vi "HOST_0505.vi"() -> ()   [LabVIEW 2018]
uses:
  <vilib>/rvi/interface/nirviMethod/nirviMethod.xnode
  <vilib>/FPGAPlugInAG/Dynamic/niLvFpga_Reset_Dynamic.vi
  <vilib>/FPGAPlugInAG/Dynamic/niLvFpga_Run_Dynamic.vi
  <vilib>/rvi/interface/nirviOpenFPGA/nirviOpenFPGA.xnode
  <vilib>/rvi/interface/nirviReadWriteControl/nirviReadWriteControl.xnode
  NiFpgaLv.dll
  <vilib>/Utility/error.llb/Error Cluster From Error Code.vi
  <vilib>/rvi/interface/Simulation/niFpgaSimulationCallBeginRW.vi
  <vilib>/rvi/errors/niLvFpgaAdjustHostInterfaceError.vi
  <vilib>/rvi/interface/nirviCloseFPGA/nirviCloseFPGA.xnode
  <instrlib>/niDCPower/nidcpower.llb/niDCPower Measurement Type.ctl
  <vilib>/FPGAPlugInAG/Dynamic/niLvFpga_ReadFifo_Dynamic.vi
  <vilib>/rvi/errors/niLvFpgaMergeErrorWithErrorCode.vi
  <vilib>/FPGAPlugInAG/Dynamic/niLvFpga_Close_Dynamic.vi
  FPGA Bitfiles/GMAX0505_FPGATarget_Target0505_42rFBjRCR8s.lvbitx
  <vilib>/FPGAPlugInAG/PXI-7953R/niLvFpga_Open_PXI-7953R.vi
  <vilib>/rvi/interface/common/dynamic/niFpgaDynamicAddResources.vi
  <vilib>/userdefined/High Color/nirio_resource_hc.ctl
panel:
  out "Прочитали":u8[](array[numeric])
  out "Регистры":bool[](array[boolean])
  in  "Регистры":u8[](array[numeric])=[35, 5, 0, 244, 1, 0, 1, 0, 0, 0, 0, 0, 34, 20, 1, 0, 0, 7, 0, 4, 0, 0, 20, 0, 0, 0, 0, 0, 0, 0, 0, 0, 0, 0, 0, 0, 0, 0, 0, 0, 0, 0, 0, 0, 0, 0, 0, 0, 0, 0, 0, 0, 0, 0, 0, 0, 0, 0, 0, 0, 0, 0, 0, 0, 0, 0, 0, 0, 0, 0, 0, 0, 0, 0, 0, 0, 0, 0, 0, 0, 0, 0, 0, 50, 20, 0, 0, 6, 2, 2, 4, 4, 0, 32, 35, 1, 196, 53, 203, 59, 53, 252, 255, 255, 255, 255, 255, 255, 255, 255, 52, 216, 16, 79, 61, 0, 8, 144, 192, 29, 9, 196, 50, 75, 91, 5, 208, 160, 195, 68, 2, 16, 112, 67, 14, 48, 208, 240, 208, 68, 7, 208, 192, 195, 68, 52, 240, 128, 195, 255, 75, 164, 161, 64, 14, 65, 252, 31, 129, 12, 124, 0, 24, 27, 1, 0, 2, 0, 5, 0, 0, 0, 7, 208, 192, 195, 68, 0, 1, 3, 0, 0, 0, 0, 0, 0, 0, 0, 0, 0, 0, 0, 0, 0, 0, 0, 0, 0, 0, 0, 0, 0, 176, 0, 27, 33, 128, 247, 131, 128, 165, 204, 119, 243, 221, 13, 211, 0, 0, 28, 176, 13, 254, 98, 193, 31, 138, 202, 231, 168, 60, 138, 254, 130, 52, 127, 193, 32, 2, 0, 0, 0, 0, 0, 0, 0, 0, 0, 0, 0, 0, 0, 0, 0, 0, 0]
  out "Записали адресов":u32
  out "世男":bool
  out "Data":u64[][](array[numeric])
  out "Image":T1(plugin-control)
  in  "Период опроса, мс":u32=1
  in  "3,3V_LVDS, V":dbl=3.3 caption="voltage level" format="%_6p"
  in  "3,3V_LVDS_curlim":dbl=0.2 caption="current limit" format="%_6p"
  out "3,3V_LVDS_char":dbl(graph)=1.5967060684808935e-06
  in  "VDDPIX, V":dbl=3.6 caption="voltage level" format="%_6p"
  in  "VDDPIX_curlim":dbl=0.3 caption="current limit" format="%_6p"
  out "VDDPIX_char":dbl(graph)=1.5967060684808935e-06
  in  "VG_RSTH, V":dbl=4.1 caption="voltage level" format="%_6p"
  in  "VG_RSTH_curlim":dbl=0.1 caption="current limit" format="%_6p"
  out "VG_RSTH_char":dbl(graph)=1.5967060684808935e-06
  in  "LED, V":dbl=-3.0 caption="voltage level" format="%_6p"
  in  "LED_curlim":dbl=0.05 caption="current limit" format="%_6p"
  out "LED_char":dbl(graph)=1.5967060684808935e-06
  in  "VDD33A, V":dbl=3.3 caption="voltage level" format="%_6p"
  in  "VDD33A_curlim":dbl=0.3 caption="current limit" format="%_6p"
  out "VDD33A_char":dbl(graph)=1.5967060684808935e-06
  in  "W(T)/R(F)":bool
  in  "Автомат":bool
  in  "VTXH, V":dbl=3.6 caption="voltage level" format="%_6p"
  in  "VDDIO, V":dbl=3.3 caption="voltage level" format="%_6p"
  in  "VDDCL, V":dbl=0.7 caption="voltage level" format="%_6p"
  in  "VDD13, V":dbl=1.3 caption="voltage level" format="%_6p"
  in  "VTXH_curlim":dbl=0.2 caption="current limit" format="%_6p"
  in  "VGRSTL_curlim":dbl=0.1 caption="current limit" format="%_6p"
  in  "VDDIO_curlim":dbl=0.1 caption="current limit" format="%_6p"
  in  "VDDCL_curlim":dbl=0.1 caption="current limit" format="%_6p"
  in  "VTXL_curlim":dbl=0.1 caption="current limit" format="%_6p"
  in  "VDD13_curlim":dbl=1.0 caption="current limit" format="%_6p"
  in  "VGRSTL, V":dbl=-1.3 caption="voltage level" format="%_6p"
  in  "VTXL, V":dbl=-1.3 caption="voltage level" format="%_6p"
  out "VTXH_char":dbl(graph)=-0.007753012065680951
  out "VGRSTL_char":dbl(graph)=6.909391540672134e-05
  out "VDDIO_char":dbl(graph)=9.424895165128459e-05
  out "VDDCL_char":dbl(graph)=-9.950040532110056e-06
  out "VTXL_char":dbl(graph)=9.067752968783287e-05
  out "VDD13_char":dbl(graph)=1.5967060684808935e-06
  in  "VDDPIX_selcur":dbl=0.2 caption="current limit" format="%_6p"
  in  "VDD33A_selcur":dbl=0.2 caption="current limit" format="%_6p"
  in  "VDD13_selcur":dbl=0.75 caption="current limit" format="%_6p"
  in  "VTXL_selcur":dbl=0.09 caption="current limit" format="%_6p"
  out "VDDCL_cur":dbl caption="measurement" format="%_6g"
  out "VTXL_cur":dbl caption="measurement" format="%_6g"
  out "VDD13_cur":dbl caption="measurement" format="%_6g"
  out "VDD33A_cur":dbl caption="measurement" format="%_6g"
  in  "SEL_Time, ms":u32=100
  in  "VG_RSTH_selcur":dbl=0.05 caption="current limit" format="%_6p"
  in  "VTXH_selcur":dbl=0.1 caption="current limit" format="%_6p"
  in  "VGRSTL_selcur":dbl=0.03 caption="current limit" format="%_6p"
  in  "VDDIO_selcur":dbl=0.03 caption="current limit" format="%_6p"
  in  "VDDCL_selcur":dbl=0.02 caption="current limit" format="%_6p"
  out "VDDPIX_cur":dbl caption="measurement" format="%_6g"
  out "VDDIO_cur":dbl caption="measurement" format="%_6g"
  out "VGRSTL_cur":dbl caption="measurement" format="%_6g"
  out "VTXH_cur":dbl caption="measurement" format="%_6g"
  out "VG_RSTH_cur":dbl caption="measurement" format="%_6g"
  out "VDDPIX":u16
  out "VDDPIX":bool
  out "VDD33A":u16
  out "VDD33A":bool
  out "VDD13":u16
  out "VDD13":bool
  out "VTXL":u16
  out "VTXL":bool
  in  "3":refnum<k15>="0" caption="1"
  in  "Проверка сбоев":bool
  out "SEU":bool
  out "SEU":u16
  in  "SPI":bool
  out "REG":bool
  in  "MOVIE":bool
  in  "FRAME!":bool
  in  "SYS_RESET_N":bool
  out "SEL":bool
  in  "SIM_SEL":bool
  out "VG_RSTH":u16
  out "VDDCL":u16
  out "VTXH":u16
  out "VDDIO":u16
  out "VGRSTL":u16
  out "VG_RSTH":bool
  out "VDDCL":bool
  out "VTXH":bool
  out "VDDIO":bool
  out "VGRSTL":bool
  in  "Стоп":bool
  in  "Питание":bool
  in  "LED":bool caption="output enabled"
  in  "0":refnum<k15>="0" caption="1"
  in  "1":refnum<k15>="0"
  in  "2":refnum<k15>="0" caption="1"
  in  "resource name 2":T2="PXI1Slot9"
  in  "SEU":path=path "C:/VPL/LabView/GSENSE2020BSI/SEU"
  in  "SEL":path=path "C:/VPL/LabView/GSENSE2020BSI/SEL"
  out "Номер образца":string="1"
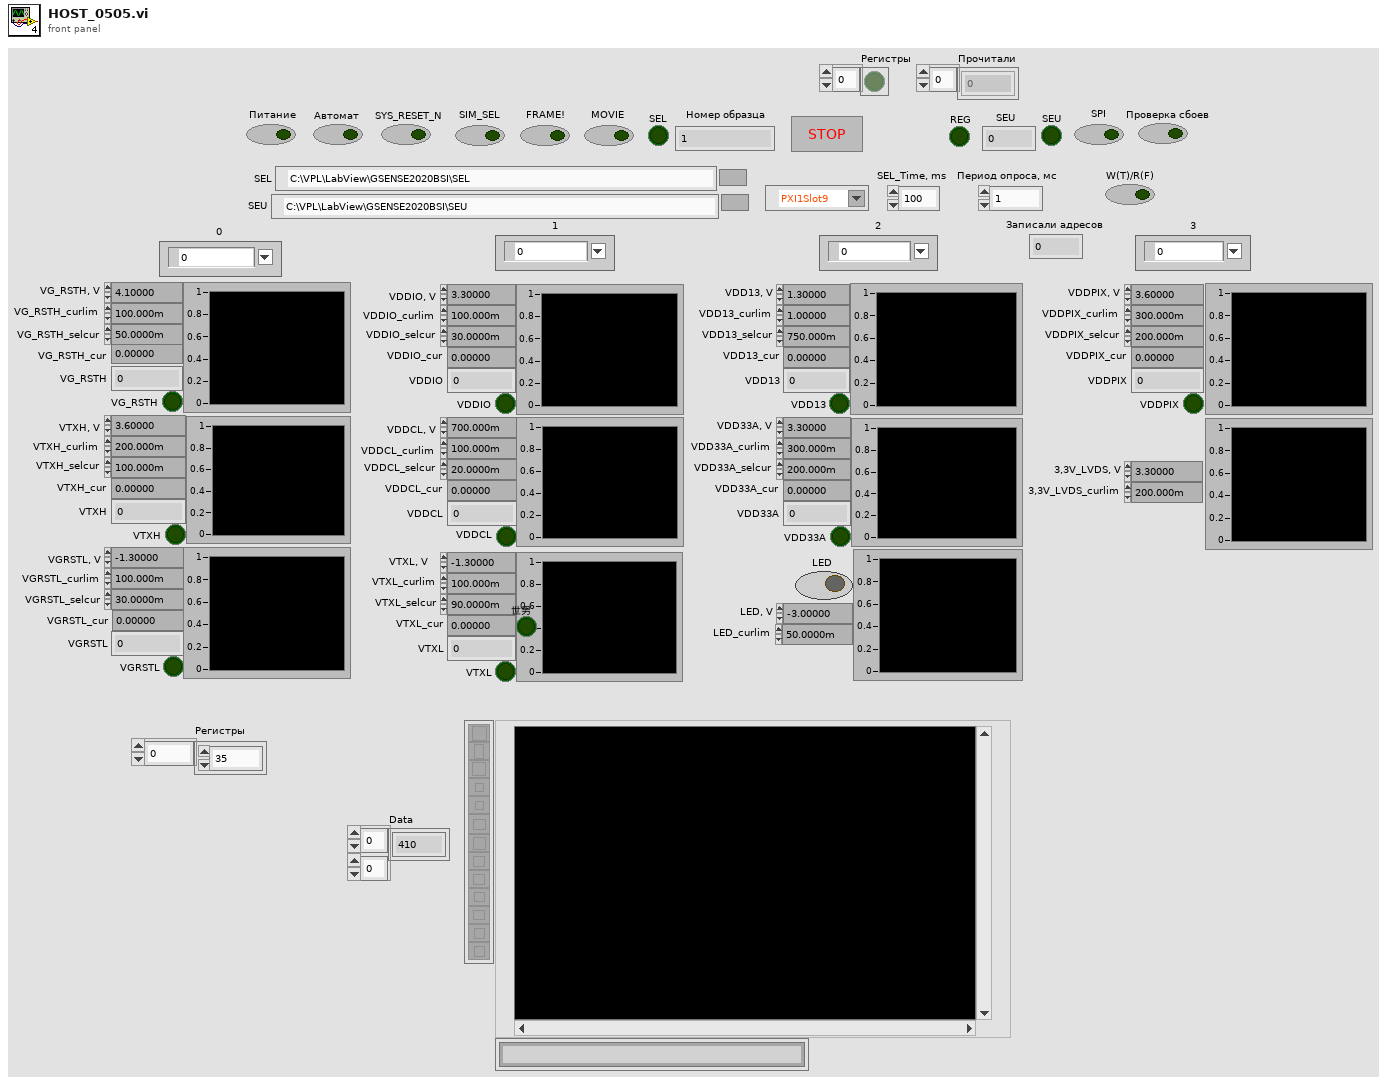
[diagram p1: front panel]
types:
  T1 = typedef "IMAQ Image.ctl" = refnum<image>
  T2 = typedef "nirio_resource_hc.ctl" = tag
  T3 = typedef "Image Type" = u32
  T4 = enum16{"open", "replace", "create", "open or create", "replace or create", "replace or create with confirmation"}
  T5 = typedef "niDCPower Measurement Type.ctl" = i32
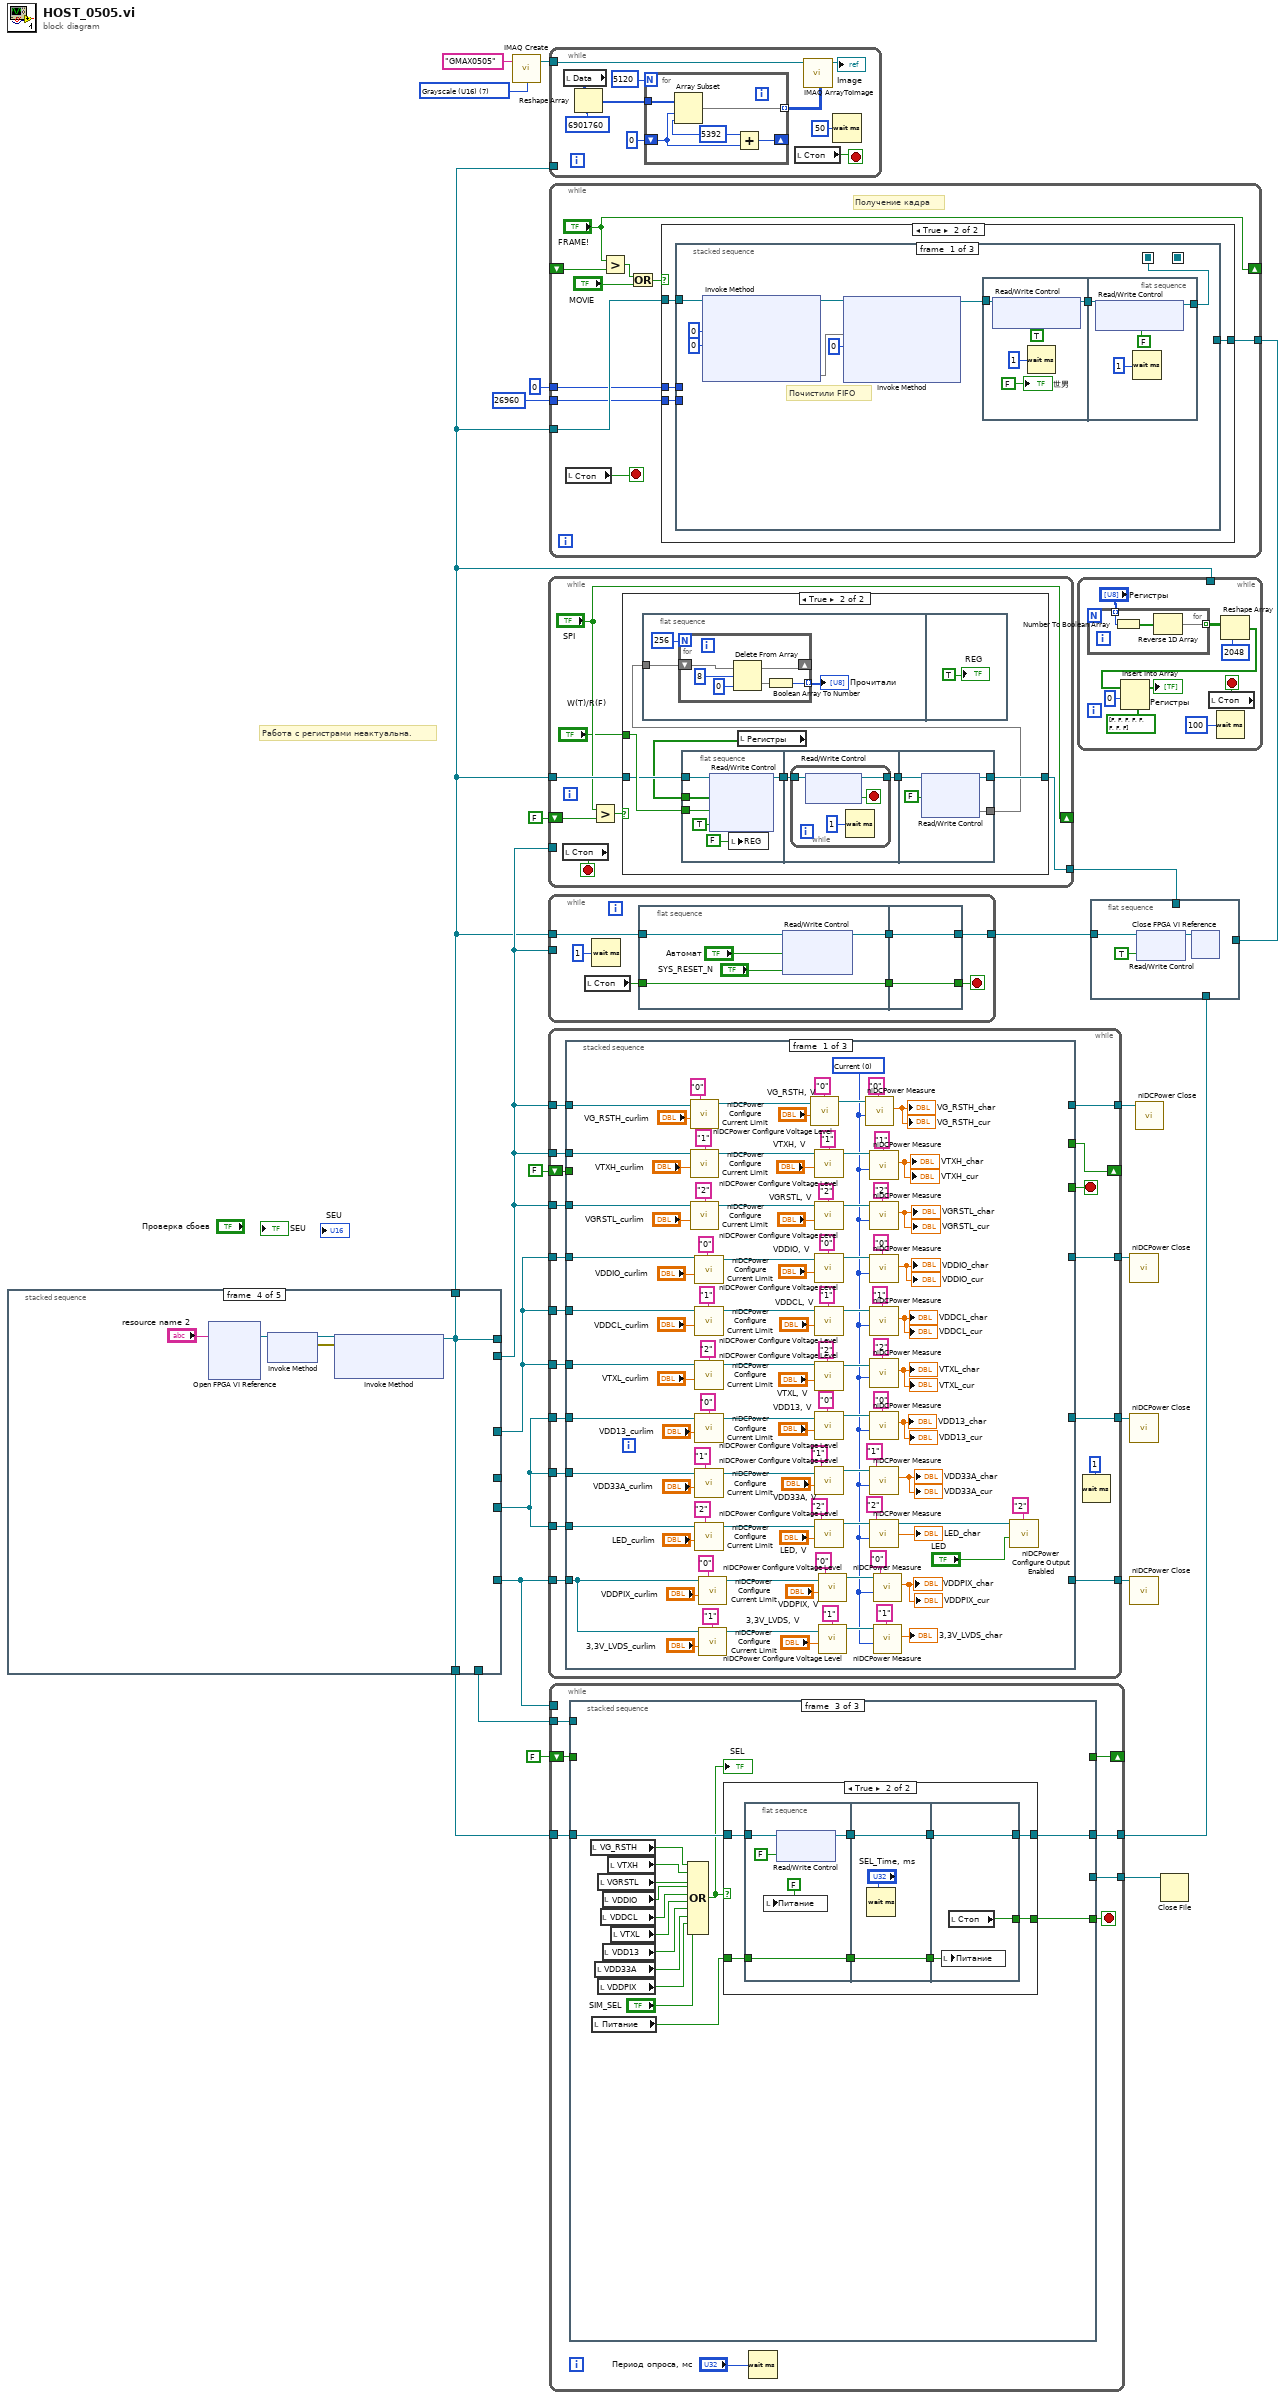
[diagram p0: block diagram]
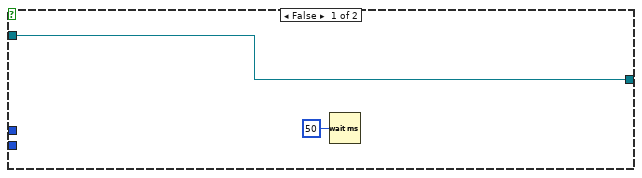
[diagram p2: hidden frame]
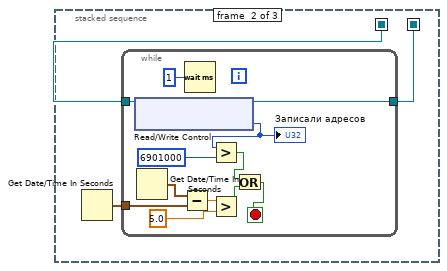
[diagram p3: hidden frame]
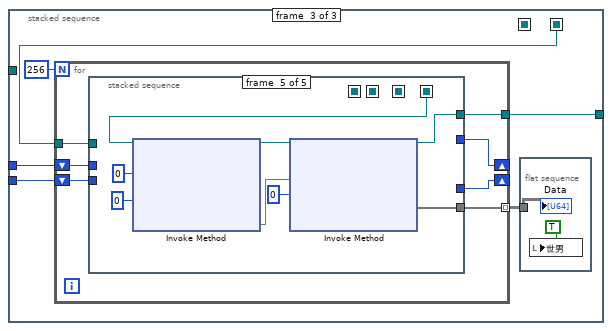
[diagram p4: hidden frame]
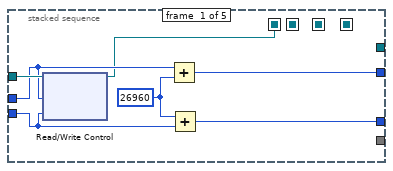
[diagram p5: hidden frame]
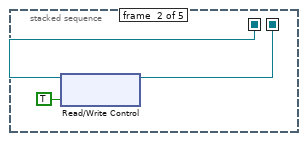
[diagram p6: hidden frame]
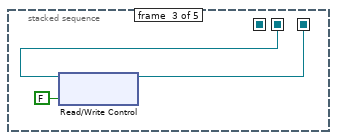
[diagram p7: hidden frame]
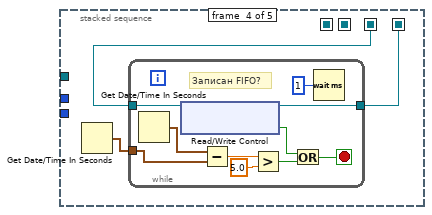
[diagram p8: hidden frame]
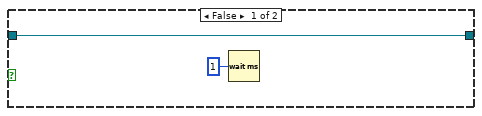
[diagram p9: hidden frame]
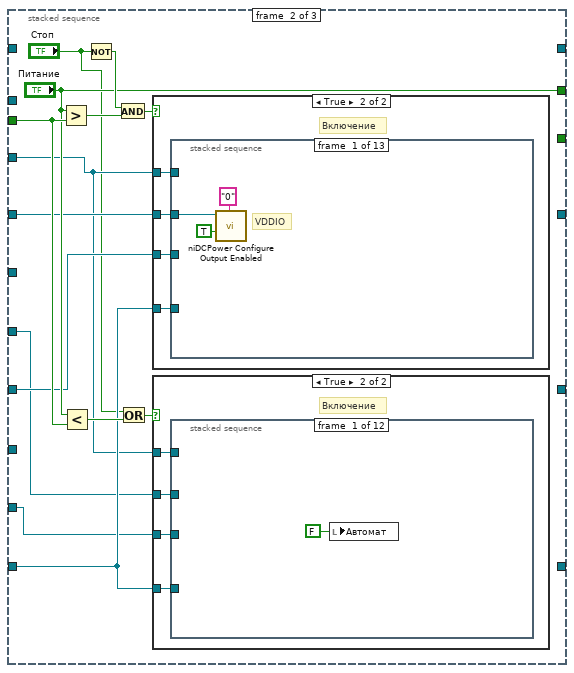
[diagram p10: hidden frame]
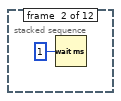
[diagram p12: hidden frame]
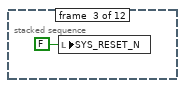
[diagram p13: hidden frame]
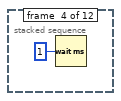
[diagram p14: hidden frame]
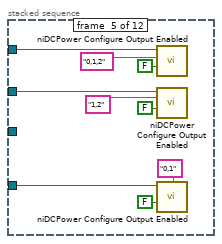
[diagram p15: hidden frame]
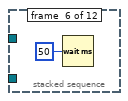
[diagram p16: hidden frame]
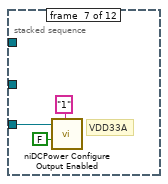
[diagram p17: hidden frame]
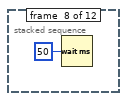
[diagram p18: hidden frame]
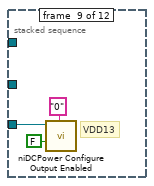
[diagram p19: hidden frame]
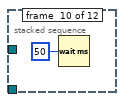
[diagram p20: hidden frame]
diagram:
  w9 = T3 7 items=["Grayscale (U8)", "Grayscale (I16)", "Grayscale (SGL)", "Complex (CSG)", "RGB (U32)", "HSL (U32)", "RGB (U64)", "Grayscale (U16)"] ("Image Type")
  # "Работа с регистрами неактуальна."
  n1 = stacked-sequence {
    tunnel: [_ _ _ _ w109] -> w17
    tunnel: [_ _ _ _ w102] -> w11
    tunnel: [_ _ _ _ w113] -> w18
    tunnel: [_ _ _ w99 _] -> w1
    tunnel: [_ _ _ w99 _] -> w21
    tunnel: [_ w36 _ _ _] -> w22
    tunnel: [_ _ w66 _ _] -> _
    tunnel: [_ _ _ w99 _] -> _
    tunnel: [_ _ _ _ w103] -> w19
    frame #0 {
      w25 = FALSE ("Стоп")
      w27 = FALSE ("Стоп")
      w28 = u16 0 ("ADC")
      # "Обнуление"
      n2 = call "Begin.vi"() -> ("Номер образца 2"=→"Номер образца":string)  [unwired: 11 in]
      n3 = local write "VTXH"(w25) -> ()
      n4 = local write "SIM_SEL"(w25) -> ()
      n5 = local write "SPI"(w25) -> ()
      n6 = local write "Проверка сбоев"(w25) -> ()
      n7 = local write "SEL"(w25) -> ()
      n8 = local write "REG"(w25) -> ()
      n9 = local write "SEU"(w28) -> ()
      n10 = local write "VTXH"(w28) -> ()
      n11 = local write "VDDCL"(w28) -> ()
      n12 = local write "VG_RSTH"(w28) -> ()
      n13 = local write "VDDIO"(w28) -> ()
      n14 = local write "VGRSTL"(w28) -> ()
      n15 = local write "SEU"(w27) -> ()
      n16 = local write "SYS_RESET_N"(w27) -> ()
      n17 = local write "Стоп"(w27) -> ()
      n18 = local write "Питание"(w27) -> ()
      n19 = local write "FRAME!"(w27) -> ()
      n20 = local write "MOVIE"(w27) -> ()
      n21 = local write "LED"(w27) -> ()
      n22 = local write "VG_RSTH"(w27) -> ()
      n23 = local write "VDDCL"(w27) -> ()
      n24 = local write "VGRSTL"(w27) -> ()
      n25 = local write "VDDIO"(w27) -> ()
    }
    frame #1 {
      w31 = "\t"
      # "Лог по токам"
      n26 = local read "Номер образца"() -> (w58:string)
      n27 = Build Path(base path="SEL", name or relative path=w58) -> (appended path=w55:path)
      n28 = Get Date/Time In Seconds() -> (seconds since 1Jan1904=w52:timestamp)
      n29 = call <vilib>:"Check if File or Folder Exists.vi"("path"=w55) -> ("file or folder exists?"=w56:bool, "dup path"=w57:path)  [unwired: 8 in, 1 out]
      n30 = Format Date/Time String(time format string (%c)="%d %H.%M.%S", seconds (now)=w52) -> (date/time string=w50:string)  [unwired: 1 in]
      n31 = case shown="False" w56 {
        tunnel: w57 -> [w64 w65]
        tunnel: [w63 w65] -> w30
        frame False {
          n32 = Create Folder(path (use dialog)=w64) -> (created path=w63:path)  [unwired: 2 in, 2 out]
        }
        frame True {
        }
      }
      n33 = Concatenate Strings(w50, ".xls" ("string")) -> (w49:string)
      n34 = Build Path(base path=w30, name or relative path=w49) -> (appended path=w51:path)
      n35 = Open/Create/Replace File(file path (use dialog)=w51, operation (0:open)=T4."open or create", access (0:read/write)=enum16{"read/write", "read-only", "write-only"}."read/write") -> (refnum out=w53:refnum<file>)  [unwired: 3 in, 2 out]
      n36 = case shown="True" TRUE {
        tunnel: w53 -> [w59 w62]
        tunnel: [w59 w60] -> w48
        frame False {
        }
        frame True {
          n37 = Set File Position(refnum=w62, from (0:start)=enum16{"start", "end", "current"}."end") -> (refnum out=w60:refnum<file>)  [unwired: 2 in, 1 out]
        }
      }
      n38 = Format Into String(initial string=w48, "Time" ("input 1"), w31, "VG_RSTH_cur", w31, "VTXH_cur", w31, "VGRSTL_cur", w31, "VDDIO_cur", w31, "VDDCL_cur", w31, "VTXL_cur", w31, "VDD13_cur", w31, "VDD33A_cur", w31, "VDDPIX_cur", w31, "\r\n") -> (resulting string=w36:refnum<file>)  [unwired: 2 in, 1 out]
    }
    frame #2 {
      w69 = "\t"
      # "Лог по сбоям"
      n39 = local read "Номер образца"() -> (w73:string)
      n40 = Build Path(base path="SEU", name or relative path=w73) -> (appended path=w87:path)
      n41 = Get Date/Time In Seconds() -> (seconds since 1Jan1904=w85:timestamp)
      n42 = call <vilib>:"Check if File or Folder Exists.vi"("path"=w87) -> ("file or folder exists?"=w88:bool, "dup path"=w89:path)  [unwired: 8 in, 1 out]
      n43 = Format Date/Time String(time format string (%c)="%d %H.%M.%S", seconds (now)=w85) -> (date/time string=w83:string)  [unwired: 1 in]
      n44 = case shown="False" w88 {
        tunnel: w89 -> [w95 w96]
        tunnel: [w94 w96] -> w74
        frame False {
          n45 = Create Folder(path (use dialog)=w95) -> (created path=w94:path)  [unwired: 2 in, 2 out]
        }
        frame True {
        }
      }
      n46 = Concatenate Strings(w83, ".xls" ("string")) -> (w82:string)
      n47 = Build Path(base path=w74, name or relative path=w82) -> (appended path=w84:path)
      n48 = Open/Create/Replace File(file path (use dialog)=w84, operation (0:open)=T4."open or create", access (0:read/write)=enum16{"read/write", "read-only", "write-only"}."read/write") -> (refnum out=w86:refnum<file>)  [unwired: 3 in, 2 out]
      n49 = case shown="True" TRUE {
        tunnel: w86 -> [w90 w93]
        tunnel: [w90 w91] -> w81
        frame False {
        }
        frame True {
          n50 = Set File Position(refnum=w93, from (0:start)=enum16{"start", "end", "current"}."end") -> (refnum out=w91:refnum<file>)  [unwired: 2 in, 1 out]
        }
      }
      n51 = Format Into String(initial string=w81, "Time" ("input 1"), w69, "Регистр №" ("input 3"), w69, "Содержание" ("input 4"), w69, "Кол-во сбоев" ("input 7"), "\r\n") -> (resulting string=w66:refnum<file>)  [unwired: 2 in, 1 out]
    }
    frame #3 {
      n52 = xnode "Open FPGA VI Reference"("resource name"="resource name 2") -> ("FPGA VI Reference Out"=w97:refnum<k20>)  [unwired: 1 in, 1 out]
      n53 = xnode "Invoke Method"("FPGA VI Reference In"=w97) -> ("FPGA VI Reference Out"=w101:refnum<k20>, "error out"=w100:errorcluster)  [unwired: 1 in]
      n54 = xnode "Invoke Method"("FPGA VI Reference In"=w101, "error in"=w100) -> ("FPGA VI Reference Out"=w99:refnum<k20>)  [unwired: 1 in, 1 out]
    }
    frame #4 {
      n55 = call <instrlib>:"niDCPower Initialize.vi"("resource name"="2") -> ("error out"=w119:errorcluster, "instrument handle out"=w116:refnum<k15>)  [unwired: 3 in, 6 out]
      n56 = call <instrlib>:"niDCPower Initialize.vi"("resource name"="1") -> ("error out"=w117:errorcluster, "instrument handle out"=w114:refnum<k15>)  [unwired: 3 in, 6 out]
      n57 = call <instrlib>:"niDCPower Initialize.vi"("resource name"="3") -> ("error out"=w107:errorcluster, "instrument handle out"=w108:refnum<k15>)  [unwired: 3 in, 6 out]
      n58 = call <instrlib>:"niDCPower Initialize.vi"("resource name"="0") -> ("error out"=w118:errorcluster, "instrument handle out"=w115:refnum<k15>)  [unwired: 3 in, 6 out]
      n59 = call <instrlib>:"niDCPower Configure Voltage Level.vi"("error in (no error)"=w119, "voltage level"=0.0, "channel name"="0,1,2", "instrument handle"=w116) -> ("instrument handle out"=w109:refnum<k15>)  [unwired: 6 in, 1 out]
      n60 = call <instrlib>:"niDCPower Configure Voltage Level.vi"("error in (no error)"=w117, "voltage level"=0.0, "channel name"="0,1,2", "instrument handle"=w114) -> ("instrument handle out"=w113:refnum<k15>)  [unwired: 6 in, 1 out]
      n61 = call <instrlib>:"niDCPower Configure Voltage Level.vi"("error in (no error)"=w107, "voltage level"=0.0, "channel name"="0,1", "instrument handle"=w108) -> ("instrument handle out"=w103:refnum<k15>)  [unwired: 6 in, 1 out]
      n62 = call <instrlib>:"niDCPower Configure Voltage Level.vi"("error in (no error)"=w118, "voltage level"=0.0, "channel name"="0,1,2", "instrument handle"=w115) -> ("instrument handle out"=w102:refnum<k15>)  [unwired: 6 in, 1 out]
    }
  }
  n63 = call "IMAQ Create"("Image Name"="GMAX0505", "Image Type"=w9) -> ("New Image"=w10:T1)  [unwired: 3 in, 1 out]
  n64 = while {
    tunnel: w1 -> [w129]
    shift-right: ["SPI"] -> _
    shift-left: FALSE ("SPI") -> [w131]
    tunnel: w11 -> [_]
    tunnel: [w127] -> w4
    stop <- w132 stop-if-true
    n65 = local read "Стоп"() -> (w132:bool)
    n66 = Greater?(x="SPI", y=w131) -> (0:w130:bool)
    n67 = case shown="True" w130 {
      tunnel: w129 -> [w133 w139]
      tunnel: [w133 w140] -> w127
      tunnel: "W(T)/R(F)" -> [_ w141]
      frame False {
        n68 = Wait (ms)(milliseconds to wait=u32 1) -> ()  [unwired: 1 out]
      }
      frame True {
        n69 = flat-sequence {
          tunnel: w135 -> [w160]
          frame #0 {
            n70 = for {
              N: 256 -> [_]
              shift-right: [w163] -> _
              shift-left: w160 -> [w166]
              tunnel: [w161] -> w158 mode=indexing
              n71 = Delete From Array(array=w166, length=8, index=0) -> (deleted portion=w162, array with subset deleted=w163)
              n72 = Boolean Array To Number(Boolean array=w162) -> (number=w161:u8)
            }
            "Прочитали" <- w158
          }
          frame #1 {
            "REG" <- TRUE ("REG")
          }
        }
        n73 = flat-sequence {
          tunnel: [w146] -> w138
          tunnel: w141 -> [w145]
          tunnel: w139 -> [w144]
          tunnel: w136 -> [w142]
          tunnel: w138 -> [w149]
          tunnel: [w148] -> w137
          tunnel: w137 -> [w157]
          tunnel: [w155] -> w140
          tunnel: [w154] -> w135
          frame #0 {
            n74 = xnode "Read/Write Control"("FPGA VI Reference In"=w144, "SPI_IN"=w142, "W(T)/R(F)"=w145, "SPI"=TRUE) -> ("FPGA VI Reference Out"=w146:refnum<k20>)  [unwired: 1 in, 1 out]
            n75 = local write "REG"(FALSE ("REG")) -> ()
          }
          frame #1 {
            n76 = while {
              tunnel: w149 -> [w153]
              tunnel: [w150] -> w148
              stop <- w152 stop-if-true
              n77 = xnode "Read/Write Control"("FPGA VI Reference In"=w153) -> ("FPGA VI Reference Out"=w150:refnum<k20>, "SPI_OFF"=w152:bool)  [unwired: 1 in, 1 out]
              n78 = Wait (ms)(milliseconds to wait=u32 1) -> ()  [unwired: 1 out]
            }
          }
          frame #2 {
            n79 = xnode "Read/Write Control"("FPGA VI Reference In"=w157, "SPI"=FALSE) -> ("FPGA VI Reference Out"=w155:refnum<k20>, "SPI_OUT"=w154)  [unwired: 1 in, 1 out]
          }
        }
        n80 = local read "Регистры"() -> (w136:bool[])
      }
    }
  }
  n81 = while {
    tunnel: w1 -> [w173]
    tunnel: [w172] -> w2
    tunnel: w11 -> [_]
    stop <- w168 stop-if-true
    n82 = local read "Стоп"() -> (w169:bool)
    n83 = Wait (ms)(milliseconds to wait=u32 1) -> ()  [unwired: 1 out]
    n84 = flat-sequence {
      tunnel: w173 -> [w179]
      tunnel: [w178] -> w171
      tunnel: [w177] -> w170
      tunnel: w169 -> [w177]
      tunnel: [w181] -> w172
      tunnel: w171 -> [w181]
      tunnel: w170 -> [w180]
      tunnel: [w180] -> w168
      frame #0 {
        n85 = xnode "Read/Write Control"("FPGA VI Reference In"=w179, "Автомат"="Автомат", "SYS_RST_N"="SYS_RESET_N") -> ("FPGA VI Reference Out"=w178:refnum<k20>)  [unwired: 1 in, 1 out]
      }
      frame #1 {
      }
    }
  }
  n86 = while {
    shift-right: [w198] -> _
    shift-left: FALSE -> [w199]
    tunnel: w11 -> [w197]
    tunnel: w18 -> [w191]
    tunnel: w17 -> [w188]
    tunnel: w19 -> [w196]
    tunnel: w11 -> [w193]
    tunnel: w11 -> [w192]
    tunnel: w18 -> [w190]
    tunnel: w18 -> [w189]
    tunnel: w17 -> [w187]
    tunnel: w17 -> [w186]
    tunnel: [w185] -> w16
    tunnel: [w184] -> w15
    tunnel: [w183] -> w14
    tunnel: [w182] -> w13
    stop <- w195 stop-if-true
    n87 = stacked-sequence {
      tunnel: w199 -> [_ w315 _]
      tunnel: [_ "Питание" _] -> w198
      tunnel: w197 -> [w211 _ w379]
      tunnel: w196 -> [w200 w306 w376]
      tunnel: [_ _ w380] -> w195
      tunnel: w193 -> [w210 _ _]
      tunnel: w192 -> [w209 w303 _]
      tunnel: w191 -> [w208 w309 w378]
      tunnel: w190 -> [w207 _ _]
      tunnel: w189 -> [w206 w304 _]
      tunnel: w188 -> [w205 w308 w377]
      tunnel: w187 -> [w204 _ _]
      tunnel: w186 -> [w203 w305 _]
      tunnel: [_ _ w379] -> w185
      tunnel: [_ _ w378] -> w184
      tunnel: [_ _ w377] -> w183
      tunnel: [_ _ w376] -> w182
      frame #0 {
        w225 = T5 0 items=["Current", "Voltage"] ("measurement type")
        n88 = call <instrlib>:"niDCPower Configure Current Limit.vi"("current limit"="VG_RSTH_curlim", "channel name"="0", "instrument handle"=w211) -> ("instrument handle out"=w242:refnum<k15>)  [unwired: 7 in, 1 out]
        n89 = call <instrlib>:"niDCPower Configure Current Limit.vi"("current limit"="VTXH_curlim", "channel name"="1", "instrument handle"=w210) -> ("instrument handle out"=w282:refnum<k15>)  [unwired: 7 in, 1 out]
        n90 = call <instrlib>:"niDCPower Configure Current Limit.vi"("current limit"="VGRSTL_curlim", "channel name"="2", "instrument handle"=w209) -> ("instrument handle out"=w283:refnum<k15>)  [unwired: 7 in, 1 out]
        n91 = call <instrlib>:"niDCPower Configure Current Limit.vi"("current limit"="VDDIO_curlim", "channel name"="0", "instrument handle"=w208) -> ("instrument handle out"=w284:refnum<k15>)  [unwired: 7 in, 1 out]
        n92 = call <instrlib>:"niDCPower Configure Current Limit.vi"("current limit"="VDDCL_curlim", "channel name"="1", "instrument handle"=w207) -> ("instrument handle out"=w285:refnum<k15>)  [unwired: 7 in, 1 out]
        n93 = call <instrlib>:"niDCPower Configure Current Limit.vi"("current limit"="VTXL_curlim", "channel name"="2", "instrument handle"=w206) -> ("instrument handle out"=w286:refnum<k15>)  [unwired: 7 in, 1 out]
        n94 = call <instrlib>:"niDCPower Configure Current Limit.vi"("current limit"="VDD13_curlim", "channel name"="0", "instrument handle"=w205) -> ("instrument handle out"=w287:refnum<k15>)  [unwired: 7 in, 1 out]
        n95 = call <instrlib>:"niDCPower Configure Current Limit.vi"("current limit"="VDD33A_curlim", "channel name"="1", "instrument handle"=w204) -> ("instrument handle out"=w255:refnum<k15>)  [unwired: 7 in, 1 out]
        n96 = call <instrlib>:"niDCPower Configure Current Limit.vi"("current limit"="LED_curlim", "channel name"="2", "instrument handle"=w203) -> ("instrument handle out"=w250:refnum<k15>)  [unwired: 7 in, 1 out]
        n97 = call <instrlib>:"niDCPower Configure Current Limit.vi"("current limit"="VDDPIX_curlim", "channel name"="0", "instrument handle"=w200) -> ("instrument handle out"=w235:refnum<k15>)  [unwired: 7 in, 1 out]
        n98 = call <instrlib>:"niDCPower Configure Current Limit.vi"("current limit"="3,3V_LVDS_curlim", "channel name"="1", "instrument handle"=w200) -> ("instrument handle out"=w230:refnum<k15>)  [unwired: 7 in, 1 out]
        n99 = call <instrlib>:"niDCPower Configure Voltage Level.vi"("voltage level"="VG_RSTH, V", "channel name"="0", "instrument handle"=w242) -> ("instrument handle out"=w245:refnum<k15>)  [unwired: 7 in, 1 out]
        n100 = call <instrlib>:"niDCPower Configure Voltage Level.vi"("voltage level"="VTXH, V", "channel name"="1", "instrument handle"=w282) -> ("instrument handle out"=w265:refnum<k15>)  [unwired: 7 in, 1 out]
        n101 = call <instrlib>:"niDCPower Configure Voltage Level.vi"("voltage level"="VGRSTL, V", "channel name"="2", "instrument handle"=w283) -> ("instrument handle out"=w264:refnum<k15>)  [unwired: 7 in, 1 out]
        n102 = call <instrlib>:"niDCPower Configure Voltage Level.vi"("voltage level"="VDDIO, V", "channel name"="0", "instrument handle"=w284) -> ("instrument handle out"=w263:refnum<k15>)  [unwired: 7 in, 1 out]
        n103 = call <instrlib>:"niDCPower Configure Voltage Level.vi"("voltage level"="VDDCL, V", "channel name"="1", "instrument handle"=w285) -> ("instrument handle out"=w262:refnum<k15>)  [unwired: 7 in, 1 out]
        n104 = call <instrlib>:"niDCPower Configure Voltage Level.vi"("voltage level"="VTXL, V", "channel name"="2", "instrument handle"=w286) -> ("instrument handle out"=w261:refnum<k15>)  [unwired: 7 in, 1 out]
        n105 = call <instrlib>:"niDCPower Configure Voltage Level.vi"("voltage level"="VDD13, V", "channel name"="0", "instrument handle"=w287) -> ("instrument handle out"=w260:refnum<k15>)  [unwired: 7 in, 1 out]
        n106 = call <instrlib>:"niDCPower Configure Voltage Level.vi"("voltage level"="VDD33A, V", "channel name"="1", "instrument handle"=w255) -> ("instrument handle out"=w258:refnum<k15>)  [unwired: 7 in, 1 out]
        n107 = call <instrlib>:"niDCPower Configure Voltage Level.vi"("voltage level"="LED, V", "channel name"="2", "instrument handle"=w250) -> ("instrument handle out"=w247:refnum<k15>)  [unwired: 7 in, 1 out]
        n108 = call <instrlib>:"niDCPower Configure Voltage Level.vi"("voltage level"="VDDPIX, V", "channel name"="0", "instrument handle"=w235) -> ("instrument handle out"=w238:refnum<k15>)  [unwired: 7 in, 1 out]
        n109 = call <instrlib>:"niDCPower Configure Voltage Level.vi"("voltage level"="3,3V_LVDS, V", "channel name"="1", "instrument handle"=w230) -> ("instrument handle out"=w227:refnum<k15>)  [unwired: 7 in, 1 out]
        n110 = call <instrlib>:"niDCPower Measure.vi"("measurement type"=w225, "channel name"="0", "instrument handle"=w245) -> ("measurement"=→"VG_RSTH_char" →"VG_RSTH_cur":dbl)  [unwired: 6 in, 2 out]
        n111 = call <instrlib>:"niDCPower Measure.vi"("measurement type"=w225, "channel name"="1", "instrument handle"=w265) -> ("measurement"=→"VTXH_char" →"VTXH_cur":dbl)  [unwired: 6 in, 2 out]
        n112 = call <instrlib>:"niDCPower Measure.vi"("measurement type"=w225, "channel name"="2", "instrument handle"=w264) -> ("measurement"=→"VGRSTL_char" →"VGRSTL_cur":dbl)  [unwired: 6 in, 2 out]
        n113 = call <instrlib>:"niDCPower Measure.vi"("measurement type"=w225, "channel name"="0", "instrument handle"=w263) -> ("measurement"=→"VDDIO_char" →"VDDIO_cur":dbl)  [unwired: 6 in, 2 out]
        n114 = call <instrlib>:"niDCPower Measure.vi"("measurement type"=w225, "channel name"="1", "instrument handle"=w262) -> ("measurement"=→"VDDCL_char" →"VDDCL_cur":dbl)  [unwired: 6 in, 2 out]
        n115 = call <instrlib>:"niDCPower Measure.vi"("measurement type"=w225, "channel name"="2", "instrument handle"=w261) -> ("measurement"=→"VTXL_char" →"VTXL_cur":dbl)  [unwired: 6 in, 2 out]
        n116 = call <instrlib>:"niDCPower Measure.vi"("measurement type"=w225, "channel name"="0", "instrument handle"=w260) -> ("measurement"=→"VDD13_char" →"VDD13_cur":dbl)  [unwired: 6 in, 2 out]
        n117 = call <instrlib>:"niDCPower Measure.vi"("measurement type"=w225, "channel name"="1", "instrument handle"=w258) -> ("measurement"=→"VDD33A_char" →"VDD33A_cur":dbl)  [unwired: 6 in, 2 out]
        n118 = call <instrlib>:"niDCPower Measure.vi"("measurement type"=w225, "channel name"="2", "instrument handle"=w247) -> ("measurement"=→"LED_char":dbl, "instrument handle out"=w213:refnum<k15>)  [unwired: 6 in, 1 out]
        n119 = call <instrlib>:"niDCPower Measure.vi"("measurement type"=w225, "channel name"="0", "instrument handle"=w238) -> ("measurement"=→"VDDPIX_char" →"VDDPIX_cur":dbl)  [unwired: 6 in, 2 out]
        n120 = call <instrlib>:"niDCPower Measure.vi"("measurement type"=w225, "channel name"="1", "instrument handle"=w227) -> ("measurement"=→"3,3V_LVDS_char":dbl)  [unwired: 6 in, 2 out]
        n121 = call <instrlib>:"niDCPower Configure Output Enabled.vi"("output enabled"="LED", "channel name"="2", "instrument handle"=w213) -> ()  [unwired: 7 in, 2 out]
      }
      frame #1 {
        n122 = Greater?(x="Питание", y=w315) -> (0:w313:bool)
        n123 = Less?(x="Питание", y=w315) -> (x < y?=w311:bool)
        n124 = Not(x="Стоп") -> (.not. x?=w312:bool)
        n125 = And(x=w312, y=w313) -> (x .and. y?=w314:bool)
        n126 = Or(x="Стоп", y=w311) -> (x .or. y?=w307:bool)
        n127 = case shown="True" w314 {
          tunnel: w309 -> [_ w349]
          tunnel: w308 -> [_ w348]
          tunnel: w303 -> [_ w347]
          tunnel: w306 -> [_ w346]
          frame False {
          }
          frame True {
            # "Включение"
            n128 = stacked-sequence {
              tunnel: w349 -> [w350 _ _ _ _ _ w366 _ _ _ _ _ _]
              tunnel: w348 -> [_ _ w354 _ w358 _ _ _ _ _ _ _ _]
              tunnel: w347 -> [_ _ _ _ _ _ w369 _ _ _ _ _ _]
              tunnel: w346 -> [_ _ _ _ _ _ w365 _ _ _ _ _ _]
              frame #0 {
                # "VDDIO"
                n129 = call <instrlib>:"niDCPower Configure Output Enabled.vi"("output enabled"=TRUE, "channel name"="0", "instrument handle"=w350) -> ()  [unwired: 7 in, 2 out]
              }
              frame #1 {
                n130 = Wait (ms)(milliseconds to wait=u32 50) -> ()  [unwired: 1 out]
              }
              frame #2 {
                # "VDD13"
                n131 = call <instrlib>:"niDCPower Configure Output Enabled.vi"("output enabled"=TRUE, "channel name"="0", "instrument handle"=w354) -> ()  [unwired: 7 in, 2 out]
              }
              frame #3 {
                n132 = Wait (ms)(milliseconds to wait=u32 50) -> ()  [unwired: 1 out]
              }
              frame #4 {
                # "VDD33А"
                n133 = call <instrlib>:"niDCPower Configure Output Enabled.vi"("output enabled"=TRUE, "channel name"="1", "instrument handle"=w358) -> ()  [unwired: 7 in, 2 out]
              }
              frame #5 {
                n134 = Wait (ms)(milliseconds to wait=u32 50) -> ()  [unwired: 1 out]
              }
              frame #6 {
                n135 = call <instrlib>:"niDCPower Configure Output Enabled.vi"("output enabled"=TRUE, "channel name"="0,1,2", "instrument handle"=w369) -> ()  [unwired: 7 in, 2 out]
                n136 = call <instrlib>:"niDCPower Configure Output Enabled.vi"("output enabled"=TRUE, "channel name"="1,2", "instrument handle"=w366) -> ()  [unwired: 7 in, 2 out]
                n137 = call <instrlib>:"niDCPower Configure Output Enabled.vi"("output enabled"=TRUE, "channel name"="0,1", "instrument handle"=w365) -> ()  [unwired: 7 in, 2 out]
              }
              frame #7 {
                n138 = Wait (ms)(milliseconds to wait=u32 50) -> ()  [unwired: 1 out]
              }
              frame #8 {
                n139 = local write "SYS_RESET_N"(TRUE ("SYS_RESET_N")) -> ()
              }
              frame #9 {
                n140 = Wait (ms)(milliseconds to wait=u32 1) -> ()  [unwired: 1 out]
              }
              frame #10 {
                n141 = local write "Автомат"(TRUE ("Автомат")) -> ()
              }
              frame #11 {
                n142 = Wait (ms)(milliseconds to wait=u32 1) -> ()  [unwired: 1 out]
              }
              frame #12 {
                # "Прошиваем регистры"
              }
            }
          }
        }
        n143 = case shown="True" w307 {
          tunnel: w304 -> [_ w319]
          tunnel: w305 -> [_ w318]
          tunnel: w303 -> [_ w317]
          tunnel: w306 -> [_ w316]
          frame False {
          }
          frame True {
            # "Включение"
            n144 = stacked-sequence {
              tunnel: w319 -> [_ _ _ _ w328 _ _ _ _ _ w342 _]
              tunnel: w318 -> [_ _ _ _ _ _ w334 _ w338 _ _ _]
              tunnel: w317 -> [_ _ _ _ w331 _ _ _ _ _ _ _]
              tunnel: w316 -> [_ _ _ _ w327 _ _ _ _ _ _ _]
              frame #0 {
                n145 = local write "Автомат"(FALSE ("Автомат")) -> ()
              }
              frame #1 {
                n146 = Wait (ms)(milliseconds to wait=u32 1) -> ()  [unwired: 1 out]
              }
              frame #2 {
                n147 = local write "SYS_RESET_N"(FALSE ("SYS_RESET_N")) -> ()
              }
              frame #3 {
                n148 = Wait (ms)(milliseconds to wait=u32 1) -> ()  [unwired: 1 out]
              }
              frame #4 {
                n149 = call <instrlib>:"niDCPower Configure Output Enabled.vi"("output enabled"=FALSE, "channel name"="0,1,2", "instrument handle"=w331) -> ()  [unwired: 7 in, 2 out]
                n150 = call <instrlib>:"niDCPower Configure Output Enabled.vi"("output enabled"=FALSE, "channel name"="1,2", "instrument handle"=w328) -> ()  [unwired: 7 in, 2 out]
                n151 = call <instrlib>:"niDCPower Configure Output Enabled.vi"("output enabled"=FALSE, "channel name"="0,1", "instrument handle"=w327) -> ()  [unwired: 7 in, 2 out]
              }
              frame #5 {
                n152 = Wait (ms)(milliseconds to wait=u32 50) -> ()  [unwired: 1 out]
              }
              frame #6 {
                # "VDD33А"
                n153 = call <instrlib>:"niDCPower Configure Output Enabled.vi"("output enabled"=FALSE, "channel name"="1", "instrument handle"=w334) -> ()  [unwired: 7 in, 2 out]
              }
              frame #7 {
                n154 = Wait (ms)(milliseconds to wait=u32 50) -> ()  [unwired: 1 out]
              }
              frame #8 {
                # "VDD13"
                n155 = call <instrlib>:"niDCPower Configure Output Enabled.vi"("output enabled"=FALSE, "channel name"="0", "instrument handle"=w338) -> ()  [unwired: 7 in, 2 out]
              }
              frame #9 {
                n156 = Wait (ms)(milliseconds to wait=u32 50) -> ()  [unwired: 1 out]
              }
              frame #10 {
                # "VDDIO"
                n157 = call <instrlib>:"niDCPower Configure Output Enabled.vi"("output enabled"=FALSE, "channel name"="0", "instrument handle"=w342) -> ()  [unwired: 7 in, 2 out]
              }
              frame #11 {
                n158 = Wait (ms)(milliseconds to wait=u32 50) -> ()  [unwired: 1 out]
              }
            }
          }
        }
      }
      frame #2 {
        n159 = local read "Стоп"() -> (w380:bool)
      }
    }
    n160 = Wait (ms)(milliseconds to wait=u32 1) -> ()  [unwired: 1 out]
  }
  n161 = while {
    tunnel: w10 -> [w387]
    tunnel: w1 -> [_]
    stop <- w390 stop-if-true
    n162 = local read "Data"() -> (w383:u64[][])
    n163 = Reshape Array(w383, 6901760 ("dimension size")) -> (w381:u64[])
    n164 = for {
      N: 5120 ("length 2") -> [_]
      tunnel: w381 -> [w395]
      shift-right: [w394] -> _
      shift-left: 0 ("index") -> [w393]
      tunnel: [w392] -> w385 mode=indexing
      w391 = 5392 ("length")
      n165 = Array Subset(array=w395, index=w393, length=w391) -> (w392:u64[])
      n166 = Add(x=w391, y=w393) -> (x+y=w394:i32)
    }
    n167 = local read "Стоп"() -> (w390:bool)
    n168 = call "IMAQ ArrayToImage"("Image Pixels (U16)"=w385, "Image"=w387) -> ("Image Out"=→"Image":T1)  [unwired: 8 in, 1 out]
    n169 = Wait (ms)(milliseconds to wait=u32 50) -> ()  [unwired: 1 out]
  }
  n170 = while {
    tunnel: w1 -> [w402]
    shift-right: ["FRAME!"] -> _
    shift-left: _ -> [w405]
    tunnel: u32 0 -> [w401]
    tunnel: u32 26960 ("163840") -> [w400]
    tunnel: [w399] -> w3
    stop <- w398 stop-if-true
    # "Получение кадра"
    n171 = local read "Стоп"() -> (w398:bool)
    n172 = Greater?(x="FRAME!", y=w405) -> (0:w404:bool)
    n173 = Or(x=w404, y="MOVIE") -> (x .or. y?=w403:bool)
    n174 = case shown="True" w403 {
      tunnel: w402 -> [w406 w411]
      tunnel: w401 -> [_ w410]
      tunnel: w400 -> [_ w409]
      tunnel: [w406 w408] -> w399
      frame False {
        n175 = Wait (ms)(milliseconds to wait=u32 50) -> ()  [unwired: 1 out]
      }
      frame True {
        n176 = stacked-sequence {
          seq-local: [w413 _ _] -> [_ w431 _]
          seq-local: [_ w430 _] -> [_ _ w446]
          tunnel: w411 -> [w416 _ _]
          tunnel: w410 -> [_ _ w449]
          tunnel: w409 -> [_ _ w448]
          tunnel: [_ _ w445] -> w408
          frame #0 {
            # "Почистили FIFO"
            n177 = xnode "Invoke Method"("FPGA VI Reference In"=w416, "Number of Elements"=u32 0, "Timeout (ms)"=0) -> ("FPGA VI Reference Out"=w415:refnum<k20>, "Elements Remaining"=w417)  [unwired: 1 in, 2 out]
            n178 = xnode "Invoke Method"("FPGA VI Reference In"=w415, "Number of Elements"=w417, "Timeout (ms)"=0) -> ("FPGA VI Reference Out"=w414:refnum<k20>)  [unwired: 1 in, 3 out]
            n179 = flat-sequence {
              tunnel: w414 -> [w425]
              tunnel: [w421] -> w412
              tunnel: [w427] -> w413
              tunnel: w412 -> [w426]
              frame #0 {
                n180 = xnode "Read/Write Control"("FPGA VI Reference In"=w425, "Кадр в память"=TRUE ("EXPOSURE")) -> ("FPGA VI Reference Out"=w421:refnum<k20>)  [unwired: 1 in, 1 out]
                n181 = Wait (ms)(milliseconds to wait=u32 1) -> ()  [unwired: 1 out]
                "世男" <- FALSE
              }
              frame #1 {
                n182 = xnode "Read/Write Control"("FPGA VI Reference In"=w426, "Кадр в память"=FALSE) -> ("FPGA VI Reference Out"=w427:refnum<k20>)  [unwired: 1 in, 1 out]
                n183 = Wait (ms)(milliseconds to wait=u32 1) -> ()  [unwired: 1 out]
              }
            }
          }
          frame #1 {
            n184 = Get Date/Time In Seconds() -> (seconds since 1Jan1904=w432:timestamp)
            n185 = while {
              tunnel: [w443] -> w430
              tunnel: w431 -> [w442]
              tunnel: w432 -> [w439]
              stop <- w434 stop-if-true
              n186 = xnode "Read/Write Control"("FPGA VI Reference In"=w442) -> ("FPGA VI Reference Out"=w443:refnum<k20>, "Записали адресов"=w433:u32)  [unwired: 1 in, 1 out]
              "Записали адресов" <- w433
              n187 = Get Date/Time In Seconds() -> (seconds since 1Jan1904=w440:timestamp)
              n188 = Subtract(x=w440, y=w439) -> (x-y=w438:dbl)
              n189 = Wait (ms)(milliseconds to wait=u32 1) -> ()  [unwired: 1 out]
              n190 = Greater?(x=w433, y=u32 6901000) -> (0:w436:bool)
              n191 = Greater?(x=w438, y=5.0) -> (0:w435:bool)
              n192 = Or(x=w436, y=w435) -> (x .or. y?=w434:bool)
            }
          }
          frame #2 {
            n193 = for {
              N: 256 -> [_]
              tunnel: w446 -> [w459]
              shift-right: [w456] -> _
              shift-left: w449 -> [w458]
              shift-right: [w455] -> _
              shift-left: w448 -> [w457]
              tunnel: [w454] -> w447 mode=indexing
              tunnel: [w453] -> w445
              n194 = stacked-sequence {
                seq-local: [w460 _ _ _ _] -> [_ w468 _ _ _]
                seq-local: [_ w467 _ _ _] -> [_ _ w471 _ _]
                seq-local: [_ _ w470 _ _] -> [_ _ _ w475 _]
                seq-local: [_ _ _ w474 _] -> [_ _ _ _ w486]
                tunnel: w459 -> [w466 _ _ _ _]
                tunnel: w458 -> [w464 _ _ _ _]
                tunnel: w457 -> [w463 _ _ _ _]
                tunnel: [w462 _ _ _ _] -> w456
                tunnel: [w461 _ _ _ _] -> w455
                tunnel: [_ _ _ _ w488] -> w454
                tunnel: [_ _ _ _ w487] -> w453
                frame #0 {
                  w465 = u32 26960 ("163840")
                  n195 = xnode "Read/Write Control"("FPGA VI Reference In"=w466, "Нач_адр"=w464, "Кон_адр"=w463) -> ("FPGA VI Reference Out"=w460:refnum<k20>)  [unwired: 1 in, 1 out]
                  n196 = Add(x=w464, y=w465) -> (x+y=w462:u32)
                  n197 = Add(x=w465, y=w463) -> (x+y=w461:u32)
                }
                frame #1 {
                  n198 = xnode "Read/Write Control"("FPGA VI Reference In"=w468, "Кадр на ПК"=TRUE ("HOST")) -> ("FPGA VI Reference Out"=w467:refnum<k20>)  [unwired: 1 in, 1 out]
                }
                frame #2 {
                  n199 = xnode "Read/Write Control"("FPGA VI Reference In"=w471, "Кадр на ПК"=FALSE ("HOST")) -> ("FPGA VI Reference Out"=w470:refnum<k20>)  [unwired: 1 in, 1 out]
                }
                frame #3 {
                  n200 = Get Date/Time In Seconds() -> (seconds since 1Jan1904=w473:timestamp)
                  n201 = while {
                    tunnel: w475 -> [w484]
                    tunnel: [w483] -> w474
                    tunnel: w473 -> [w481]
                    stop <- w476 stop-if-true
                    # "Записан FIFO?"
                    n202 = Get Date/Time In Seconds() -> (seconds since 1Jan1904=w482:timestamp)
                    n203 = xnode "Read/Write Control"("FPGA VI Reference In"=w484) -> ("FPGA VI Reference Out"=w483:refnum<k20>, "Записали FIFO"=w478:bool)  [unwired: 1 in, 1 out]
                    n204 = Subtract(x=w482, y=w481) -> (x-y=w480:dbl)
                    n205 = Greater?(x=w480, y=5.0) -> (0:w477:bool)
                    n206 = Or(x=w478, y=w477) -> (x .or. y?=w476:bool)
                    n207 = Wait (ms)(milliseconds to wait=u32 1) -> ()  [unwired: 1 out]
                  }
                }
                frame #4 {
                  n208 = xnode "Invoke Method"("FPGA VI Reference In"=w486, "Number of Elements"=u32 0, "Timeout (ms)"=0) -> ("FPGA VI Reference Out"=w492:refnum<k20>, "Elements Remaining"=w493)  [unwired: 1 in, 2 out]
                  n209 = xnode "Invoke Method"("FPGA VI Reference In"=w492, "Number of Elements"=w493, "Timeout (ms)"=0) -> ("FPGA VI Reference Out"=w487:refnum<k20>, "Data"=w488:void[])  [unwired: 1 in, 2 out]
                }
              }
            }
            n210 = flat-sequence {
              tunnel: w447 -> [w451]
              frame #0 {
                n211 = local write "世男"(TRUE) -> ()
                "Data" <- w451
              }
            }
          }
        }
      }
    }
  }
  n212 = while {
    tunnel: w21 -> [w496]
    shift-right: [w500] -> _
    shift-left: FALSE ("Питание") -> [w501]
    tunnel: w22 -> [w498]
    tunnel: [w495] -> w23
    tunnel: [w494] -> w5
    tunnel: w19 -> [_]
    stop <- w497 stop-if-true
    n213 = stacked-sequence {
      tunnel: w501 -> [w504 _ _]
      tunnel: [w503 _ _] -> w500
      tunnel: w498 -> [_ w605 _]
      tunnel: [_ _ w625] -> w497
      tunnel: w496 -> [_ _ w624]
      tunnel: [_ w594 _] -> w495
      tunnel: [_ _ w622] -> w494
      frame #0 {
        n214 = flat-sequence {
          tunnel: w502 -> [w505]
          frame #0 {
            n215 = case shown="True" w505 {
              frame False {
              }
              frame True {
                n216 = Wait (ms)(milliseconds to wait=u32 500) -> ()  [unwired: 1 out]
              }
            }
          }
          frame #1 {
            n217 = local read "VG_RSTH_cur"() -> (w526:dbl)
            n218 = local read "VTXH_cur"() -> (w527:dbl)
            n219 = local read "VGRSTL_cur"() -> (w528:dbl)
            n220 = local read "VDDIO_cur"() -> (w529:dbl)
            n221 = local read "VDDCL_cur"() -> (w520:dbl)
            n222 = local read "VTXL_cur"() -> (w519:dbl)
            n223 = local read "VDD13_cur"() -> (w518:dbl)
            n224 = local read "VDD33A_cur"() -> (w517:dbl)
            n225 = local read "VDDPIX_cur"() -> (w516:dbl)
            n226 = Greater Or Equal?(x=w516, y="VDDPIX_selcur") -> (x >= y?=w507:bool)
            "VDDPIX" <- w507
            n227 = Greater Or Equal?(x=w519, y="VTXL_selcur") -> (x >= y?=w510:bool)
            "VTXL" <- w510
            n228 = Greater Or Equal?(x=w517, y="VDD33A_selcur") -> (x >= y?=w508:bool)
            "VDD33A" <- w508
            n229 = Greater Or Equal?(x=w527, y="VTXH_selcur") -> (x >= y?=w514:bool)
            "VTXH" <- w514
            n230 = Greater Or Equal?(x=w520, y="VDDCL_selcur") -> (x >= y?=w511:bool)
            "VDDCL" <- w511
            n231 = Greater Or Equal?(x=w518, y="VDD13_selcur") -> (x >= y?=w509:bool)
            "VDD13" <- w509
            n232 = Greater Or Equal?(x=w526, y="VG_RSTH_selcur") -> (x >= y?=w515:bool)
            "VG_RSTH" <- w515
            n233 = Greater Or Equal?(x=w528, y="VGRSTL_selcur") -> (x >= y?=w513:bool)
            "VGRSTL" <- w513
            n234 = Greater Or Equal?(x=w529, y="VDDIO_selcur") -> (x >= y?=w512:bool)
            "VDDIO" <- w512
            n235 = case shown="True" w515 {
              frame False {
              }
              frame True {
                n236 = local read "VG_RSTH"() -> (w550:u16)
                n237 = Increment(x=w550) -> (x+1=→"VG_RSTH":u16)
              }
            }
            n238 = case shown="True" w513 {
              frame False {
              }
              frame True {
                n239 = local read "VGRSTL"() -> (w546:u16)
                n240 = Increment(x=w546) -> (x+1=→"VGRSTL":u16)
              }
            }
            n241 = case shown="True" w512 {
              frame False {
              }
              frame True {
                n242 = local read "VDDIO"() -> (w544:u16)
                n243 = Increment(x=w544) -> (x+1=→"VDDIO":u16)
              }
            }
            n244 = case shown="True" w514 {
              frame False {
              }
              frame True {
                n245 = local read "VTXH"() -> (w548:u16)
                n246 = Increment(x=w548) -> (x+1=→"VTXH":u16)
              }
            }
            n247 = case shown="True" w511 {
              frame False {
              }
              frame True {
                n248 = local read "VDDCL"() -> (w542:u16)
                n249 = Increment(x=w542) -> (x+1=→"VDDCL":u16)
              }
            }
            n250 = case shown="True" w510 {
              frame False {
              }
              frame True {
                n251 = local read "VTXL"() -> (w540:u16)
                n252 = Increment(x=w540) -> (x+1=→"VTXL":u16)
              }
            }
            n253 = case shown="True" w509 {
              frame False {
              }
              frame True {
                n254 = local read "VDD13"() -> (w538:u16)
                n255 = Increment(x=w538) -> (x+1=→"VDD13":u16)
              }
            }
            n256 = case shown="True" w508 {
              frame False {
              }
              frame True {
                n257 = local read "VDD33A"() -> (w536:u16)
                n258 = Increment(x=w536) -> (x+1=→"VDD33A":u16)
              }
            }
            n259 = case shown="True" w507 {
              frame False {
              }
              frame True {
                n260 = local read "VDDPIX"() -> (w534:u16)
                n261 = Increment(x=w534) -> (x+1=→"VDDPIX":u16)
              }
            }
          }
        }
        n262 = local read "Питание"() -> (w503:bool)
        n263 = Greater?(x=w503, y=w504) -> (0:w502:bool)
      }
      frame #1 {
        w576 = "\t"
        w592 = i16 0 ("width (-)")
        w593 = i16 3 ("width (-)")
        n264 = local read "VG_RSTH_cur"() -> (w604:dbl)
        n265 = local read "VTXH_cur"() -> (w603:dbl)
        n266 = local read "VGRSTL_cur"() -> (w595:dbl)
        n267 = local read "VDDIO_cur"() -> (w591:dbl)
        n268 = local read "VDDCL_cur"() -> (w590:dbl)
        n269 = local read "VTXL_cur"() -> (w589:dbl)
        n270 = local read "VDD13_cur"() -> (w588:dbl)
        n271 = local read "VDD33A_cur"() -> (w587:dbl)
        n272 = local read "VDDPIX_cur"() -> (w586:dbl)
        n273 = local read "VG_RSTH"() -> (w585:u16)
        n274 = local read "VTXH"() -> (w584:u16)
        n275 = local read "VGRSTL"() -> (w583:u16)
        n276 = local read "VDDIO"() -> (w582:u16)
        n277 = local read "VDDCL"() -> (w581:u16)
        n278 = local read "VTXL"() -> (w580:u16)
        n279 = local read "VDD13"() -> (w579:u16)
        n280 = local read "VDD33A"() -> (w578:u16)
        n281 = local read "VDDPIX"() -> (w577:u16)
        n282 = Get Date/Time In Seconds() -> (seconds since 1Jan1904=w610:timestamp)
        n283 = Format Date/Time String(time format string (%c)="%d %H:%M:%S:%3u", seconds (now)=w610) -> (date/time string=w602:string)  [unwired: 1 in]
        n284 = Number To Fractional String(number=w604, width (-)=w593, precision (6)=w593) -> (F-format string=w601:string)  [unwired: 1 in]
        n285 = Number To Fractional String(number=w603, width (-)=w593, precision (6)=w593) -> (F-format string=w600:string)  [unwired: 1 in]
        n286 = Number To Fractional String(number=w595, width (-)=w593, precision (6)=w593) -> (F-format string=w599:string)  [unwired: 1 in]
        n287 = Number To Fractional String(number=w591, width (-)=w593, precision (6)=w593) -> (F-format string=w598:string)  [unwired: 1 in]
        n288 = Number To Fractional String(number=w590, width (-)=w593, precision (6)=w593) -> (F-format string=w597:string)  [unwired: 1 in]
        n289 = Number To Fractional String(number=w589, width (-)=w593, precision (6)=w593) -> (F-format string=w575:string)  [unwired: 1 in]
        n290 = Number To Fractional String(number=w588, width (-)=w593, precision (6)=w593) -> (F-format string=w574:string)  [unwired: 1 in]
        n291 = Number To Fractional String(number=w587, width (-)=w593, precision (6)=w593) -> (F-format string=w573:string)  [unwired: 1 in]
        n292 = Number To Fractional String(number=w586, width (-)=w593, precision (6)=w593) -> (F-format string=w572:string)  [unwired: 1 in]
        n293 = Number To Fractional String(number=w585, width (-)=w592, precision (6)=w592) -> (F-format string=w571:string)  [unwired: 1 in]
        n294 = Number To Fractional String(number=w584, width (-)=w592, precision (6)=w592) -> (F-format string=w570:string)  [unwired: 1 in]
        n295 = Number To Fractional String(number=w583, width (-)=w592, precision (6)=w592) -> (F-format string=w569:string)  [unwired: 1 in]
        n296 = Number To Fractional String(number=w582, width (-)=w592, precision (6)=w592) -> (F-format string=w568:string)  [unwired: 1 in]
        n297 = Number To Fractional String(number=w581, width (-)=w592, precision (6)=w592) -> (F-format string=w567:string)  [unwired: 1 in]
        n298 = Number To Fractional String(number=w580, width (-)=w592, precision (6)=w592) -> (F-format string=w566:string)  [unwired: 1 in]
        n299 = Number To Fractional String(number=w579, width (-)=w592, precision (6)=w592) -> (F-format string=w565:string)  [unwired: 1 in]
        n300 = Number To Fractional String(number=w578, width (-)=w592, precision (6)=w592) -> (F-format string=w564:string)  [unwired: 1 in]
        n301 = Number To Fractional String(number=w577, width (-)=w592, precision (6)=w592) -> (F-format string=w563:string)  [unwired: 1 in]
        n302 = local read "VG_RSTH"() -> (w560:bool)
        n303 = local read "VDD33A"() -> (w553:bool)
        n304 = local read "VGRSTL"() -> (w558:bool)
        n305 = local read "VDDPIX"() -> (w552:bool)
        n306 = local read "VDDCL"() -> (w556:bool)
        n307 = local read "VDDIO"() -> (w557:bool)
        n308 = local read "VDD13"() -> (w554:bool)
        n309 = local read "VTXH"() -> (w559:bool)
        n310 = local read "VTXL"() -> (w555:bool)
        n311 = Compound Arithmetic op=OR(w560, w559, w558, w557, w556, w555, w554, w553, w552) -> (w596:bool)
        n312 = Select(t="!!!", s=w596, f="") -> (s? t:f=w562:string)
        n313 = Concatenate Strings(w602, w576, w601, w576, w600, w576, w599, w576, w598, w576, w597, w576, w575, w576, w574, w576, w573, w576, w572, w576, w571, w576, w570, w576, w569, w576, w568, w576, w567, w576, w566, w576, w565, w576, w564, w576, w563, w576, w562, "\r\n") -> (w606:string)
        n314 = Format Into String(initial string=w605, w606) -> (resulting string=w594:refnum<file>)  [unwired: 2 in, 1 out]
      }
      frame #2 {
        n315 = local read "VG_RSTH"() -> (w620:bool)
        n316 = local read "Питание"() -> (w623:bool)
        n317 = local read "VDD33A"() -> (w613:bool)
        n318 = local read "VGRSTL"() -> (w618:bool)
        n319 = local read "VDDPIX"() -> (w612:bool)
        n320 = local read "VDDCL"() -> (w616:bool)
        n321 = local read "VDDIO"() -> (w617:bool)
        n322 = local read "VDD13"() -> (w614:bool)
        n323 = local read "VTXH"() -> (w619:bool)
        n324 = local read "VTXL"() -> (w615:bool)
        n325 = Compound Arithmetic op=OR(w620, w619, w618, w617, w616, w615, w614, w613, w612, "SIM_SEL") -> (w621:bool)
        "SEL" <- w621
        n326 = case shown="True" w621 {
          tunnel: [w627 w635] -> w625
          tunnel: w624 -> [w626 w634]
          tunnel: w623 -> [_ w631]
          tunnel: [w626 w630] -> w622
          frame False {
            n327 = local read "Стоп"() -> (w627:bool)
          }
          frame True {
            n328 = flat-sequence {
              tunnel: w634 -> [w639]
              tunnel: [w637] -> w632
              tunnel: w631 -> [w637]
              tunnel: [w636] -> w628
              tunnel: [w642] -> w633
              tunnel: w632 -> [w642]
              tunnel: [w641] -> w629
              tunnel: w628 -> [w641]
              tunnel: [w646] -> w635
              tunnel: w633 -> [w645]
              tunnel: [w644] -> w630
              tunnel: w629 -> [w644]
              frame #0 {
                n329 = local write "Питание"(FALSE ("Питание")) -> ()
                n330 = xnode "Read/Write Control"("FPGA VI Reference In"=w639, "Автомат"=FALSE ("Линейки")) -> ("FPGA VI Reference Out"=w636:refnum<k20>)  [unwired: 1 in, 1 out]
              }
              frame #1 {
                n331 = Wait (ms)(milliseconds to wait="SEL_Time, ms") -> ()  [unwired: 1 out]
              }
              frame #2 {
                n332 = local write "Питание"(w645) -> ()
                n333 = local read "Стоп"() -> (w646:bool)
              }
            }
          }
        }
      }
    }
    n334 = Wait (ms)(milliseconds to wait="Период опроса, мс") -> ()  [unwired: 1 out]
  }
  n335 = while {
    tunnel: w1 -> [_]
    stop <- w655 stop-if-true
    n336 = for {
      tunnel: "Регистры" -> [w658] mode=indexing
      tunnel: [w657] -> w652 mode=indexing
      n337 = Number To Boolean Array(number=w658) -> (Boolean array=w656:bool[])
      n338 = Reverse 1D Array(array=w656) -> (reversed array=w657:bool[])
    }
    n339 = local read "Стоп"() -> (w655:bool)
    n340 = Wait (ms)(milliseconds to wait=u32 100) -> ()  [unwired: 1 out]
    n341 = Reshape Array(w652, 2048 ("dimension size")) -> (w650:bool[])
    n342 = Insert Into Array(array=w650, index=0, new element=bool[] [FALSE, FALSE, FALSE, FALSE, FALSE, FALSE, FALSE, FALSE]) -> (→"Регистры":bool[])
  }
  n343 = flat-sequence {
    tunnel: w5 -> [_]
    tunnel: w4 -> [_]
    tunnel: w3 -> [_]
    tunnel: w2 -> [w660]
    frame #0 {
      n344 = xnode "Read/Write Control"("FPGA VI Reference In"=w660, "Стоп"=TRUE) -> ("FPGA VI Reference Out"=w661:refnum<k20>)  [unwired: 1 in, 1 out]
      n345 = xnode "Close FPGA VI Reference"("FPGA VI Reference In"=w661) -> ()  [unwired: 1 in, 1 out]
    }
  }
  n346 = call <instrlib>:"niDCPower Close.vi"("instrument handle"=w15) -> ()  [unwired: 10 in, 1 out]
  n347 = call <instrlib>:"niDCPower Close.vi"("instrument handle"=w14) -> ()  [unwired: 10 in, 1 out]
  n348 = call <instrlib>:"niDCPower Close.vi"("instrument handle"=w13) -> ()  [unwired: 10 in, 1 out]
  n349 = call <instrlib>:"niDCPower Close.vi"("instrument handle"=w16) -> ()  [unwired: 10 in, 1 out]
  n350 = Close File(refnum=w23) -> ()  [unwired: 1 in, 2 out]
